vi "Read_BP4610.vi"(8 "error in (no error)":errorcluster, 11 "VISAsession":refnum<visa-resource-name>) -> (0 "error out":errorcluster, 2 "Data":dbl[](array[numeric]), 3 "CopyVISAsession":refnum<visa-resource-name>)   [LabVIEW 2019]
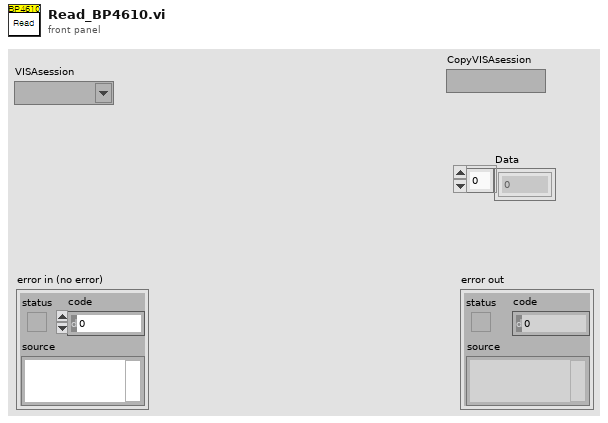
[diagram p1: front panel]
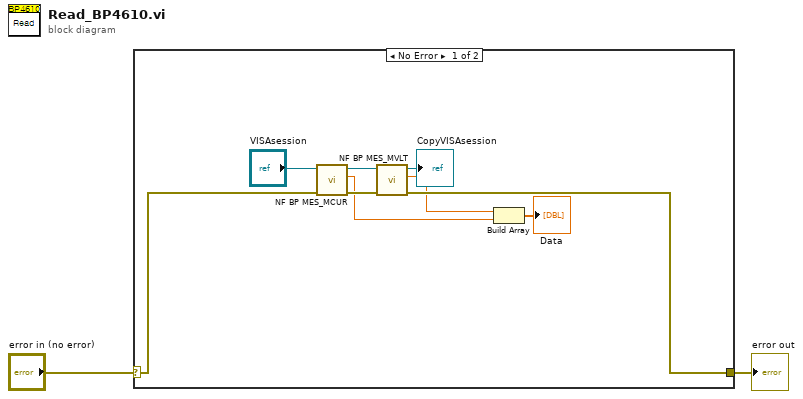
[diagram p0: block diagram]
diagram:
  n1 = case shown="No Error" "error in (no error)" {
    selector: "error in (no error)" -> [w9 w12]
    tunnel: [w8 w12] -> w1
    frame No Error {
      n2 = call <instrlib>:"NF BP MES_MCUR.vi"("error in (no error)"=w9, "VISAsession"="VISAsession") -> ("error out"=w11:errorcluster, "Query[A]"=w6:dbl, "CopyVISAsession"=w10:refnum<visa-resource-name>)  [unwired: 5 in, 2 out]
      n3 = call <instrlib>:"NF BP MES_MVLT.vi"("error in (no error)"=w11, "VISAsession"=w10) -> ("error out"=w8:errorcluster, "Query[V]"=w7:dbl, "CopyVISAsession"=→"CopyVISAsession":refnum<visa-resource-name>)  [unwired: 5 in, 2 out]
      n4 = Build Array(w7, w6) -> (→"Data":dbl[])
    }
    frame Error {
    }
  }
  "error out" <- w1
